vi "clean_up_instruments (SubVI).vi"(11 "instrum out":T1) -> ()   [LabVIEW 2016]
uses:
  <instrlib>/Agilent 33XXX Series/Agilent 33XXX Series.lvlib
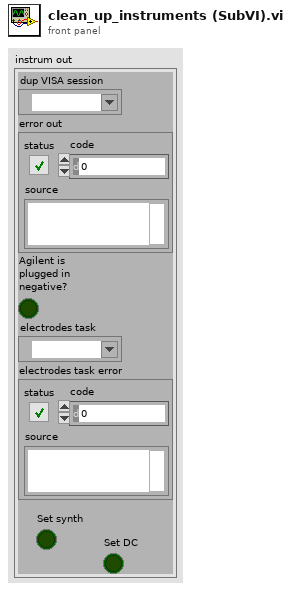
[diagram p1: front panel]
types:
  T1 = cluster{"dup VISA session":refnum<visa-resource-name>, "error out":errorcluster, "Agilent is \nplugged in \nnegative?":bool, "electrodes task":refnum<k21>, "electrodes task error":errorcluster, "Set synth":bool, "Set DC":bool}
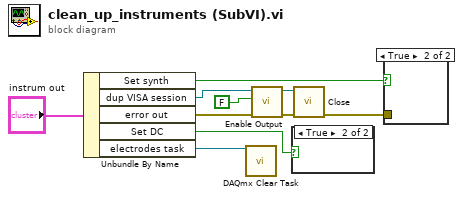
[diagram p0: block diagram]
diagram:
  n1 = Unbundle By Name("instrum out") -> ("Set synth"=w9:bool, "dup VISA session"=w6:refnum<visa-resource-name>, "error out"=w7:errorcluster, "Set DC"=w8:bool, "electrodes task"=w1:refnum<k21>)
  n2 = call <vilib>:"DAQmx Clear Task.vi"("task in"=w1) -> ()  [unwired: 14 in, 1 out]
  n3 = call <instrlib>:"Enable Output.vi"("error in (no error)"=w7, "Enable Output  (T: Enable)"=FALSE, "VISA resource name"=w6) -> ("error out"=w3:errorcluster, "VISA resource name out"=w4:refnum<visa-resource-name>)  [unwired: 7 in]
  n4 = case shown="True" w8 {
    frame False {
    }
    frame True {
    }
  }
  n5 = call <instrlib>:"Close.vi"("error in (no error)"=w3, "VISA resource name"=w4) -> ("error out"=w2:errorcluster)  [unwired: 9 in]
  n6 = case shown="True" w9 {
    tunnel: w2 -> [_ _]
    frame False {
    }
    frame True {
    }
  }
